vi "Get Wheel Type from String.vi"(10 "dvr (F)":bool, 11 "wheel type":string) -> (3 "data type":variant)   [LabVIEW 2017, in "NI_Robotics_Steering Class Types.lvlib"]
uses:
  <vilib>/robotics/Steering/Class Type Definitions/NI_Robotics_Steering Class Types.lvlib
  <vilib>/robotics/Steering/Class Type Definitions/Wheel.ctl
  <vilib>/robotics/Steering/Wheel/NI_Robotics_Wheel.lvclass
  <vilib>/robotics/Steering/Class Type Definitions/Wheel DVR.ctl
  <vilib>/robotics/Steering/Class Type Definitions/Fixed Wheel.ctl
  <vilib>/robotics/Steering/Fixed Wheel/NI_Robotics_Fixed Wheel.lvclass
  <vilib>/robotics/Steering/Class Type Definitions/Fixed Wheel DVR.ctl
  <vilib>/robotics/Steering/Class Type Definitions/Steering Wheel.ctl
  <vilib>/robotics/Steering/Steering Wheel/NI_Robotics_Steering Wheel.lvclass
  <vilib>/robotics/Steering/Class Type Definitions/Steering Wheel DVR.ctl
  <vilib>/robotics/Steering/Class Type Definitions/Caster Wheel.ctl
  <vilib>/robotics/Steering/Caster Wheel/NI_Robotics_Caster Wheel.lvclass
  <vilib>/robotics/Steering/Class Type Definitions/Caster Wheel DVR.ctl
  <vilib>/robotics/Steering/Class Type Definitions/Mecanum Wheel.ctl
  <vilib>/robotics/Steering/Mecanum Wheel/NI_Robotics_Mecanum Wheel.lvclass
  <vilib>/robotics/Steering/Class Type Definitions/Mecanum Wheel DVR.ctl
  <vilib>/robotics/Steering/Class Type Definitions/Omnidirectional Wheel.ctl
  <vilib>/robotics/Steering/Omnidirectional Wheel/NI_Robotics_Omnidirectional Wheel.lvclass
  <vilib>/robotics/Steering/Class Type Definitions/Omnidirectional Wheel DVR.ctl
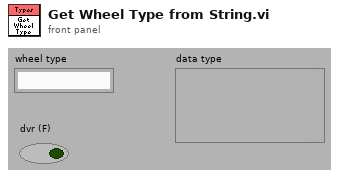
[diagram p1: front panel]
types:
  T1 = typedef "NI_Robotics_Steering Class Types.lvlib/Wheel.ctl" = refnum<class "NI_Robotics_Wheel.lvclass">
  T2 = typedef "NI_Robotics_Steering Class Types.lvlib/Wheel DVR.ctl" = refnum<data-value>
  T3 = typedef "NI_Robotics_Steering Class Types.lvlib/Fixed Wheel.ctl" = refnum<class "NI_Robotics_Fixed Wheel.lvclass">
  T4 = typedef "NI_Robotics_Steering Class Types.lvlib/Fixed Wheel DVR.ctl" = refnum<data-value>
  T5 = typedef "NI_Robotics_Steering Class Types.lvlib/Steering Wheel.ctl" = refnum<class "NI_Robotics_Steering Wheel.lvclass">
  T6 = typedef "NI_Robotics_Steering Class Types.lvlib/Steering Wheel DVR.ctl" = refnum<data-value>
  T7 = typedef "NI_Robotics_Steering Class Types.lvlib/Caster Wheel.ctl" = refnum<class "NI_Robotics_Caster Wheel.lvclass">
  T8 = typedef "NI_Robotics_Steering Class Types.lvlib/Caster Wheel DVR.ctl" = refnum<data-value>
  T9 = typedef "NI_Robotics_Steering Class Types.lvlib/Mecanum Wheel.ctl" = refnum<class "NI_Robotics_Mecanum Wheel.lvclass">
  T10 = typedef "NI_Robotics_Steering Class Types.lvlib/Mecanum Wheel DVR.ctl" = refnum<data-value>
  T11 = typedef "NI_Robotics_Steering Class Types.lvlib/Omnidirectional Wheel.ctl" = refnum<class "NI_Robotics_Omnidirectional Wheel.lvclass">
  T12 = typedef "NI_Robotics_Steering Class Types.lvlib/Omnidirectional Wheel DVR.ctl" = refnum<data-value>
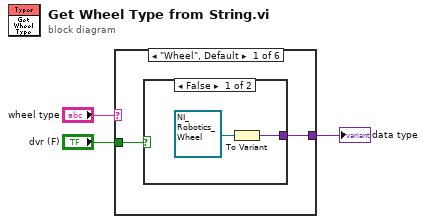
[diagram p0: block diagram]
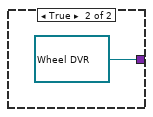
[diagram p2: hidden frame]
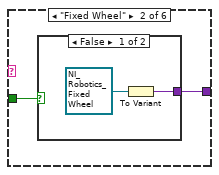
[diagram p3: hidden frame]
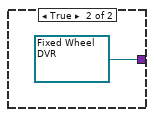
[diagram p4: hidden frame]
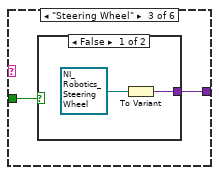
[diagram p5: hidden frame]
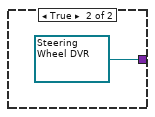
[diagram p6: hidden frame]
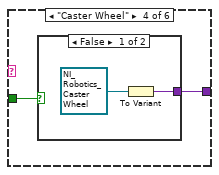
[diagram p7: hidden frame]
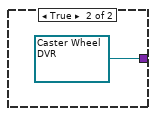
[diagram p8: hidden frame]
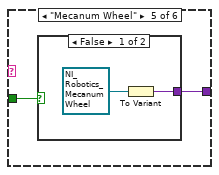
[diagram p9: hidden frame]
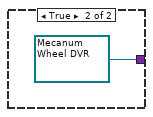
[diagram p10: hidden frame]
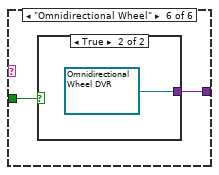
[diagram p11: hidden frame]
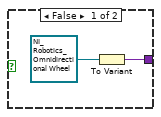
[diagram p12: hidden frame]
diagram:
  n1 = case shown="\"Wheel\", Default" "wheel type" {
    tunnel: "dvr (F)" -> [w5 w10 w15 w20 w25 w30]
    tunnel: [w4 w9 w14 w19 w24 w29] -> w1
    frame "Wheel", Default {
      n2 = case shown="False" w5 {
        tunnel: [w7 T2 refnum ("wheel ref")] -> w4
        frame False {
          n3 = To Variant(anything=T1 refnum ("wheel")) -> (Variant=w7:variant)
        }
        frame True {
        }
      }
    }
    frame "Fixed Wheel" {
      n4 = case shown="False" w10 {
        tunnel: [w12 T4 refnum ("fixed wheel ref")] -> w9
        frame False {
          n5 = To Variant(anything=T3 refnum ("fixed wheel")) -> (Variant=w12:variant)
        }
        frame True {
        }
      }
    }
    frame "Steering Wheel" {
      n6 = case shown="False" w15 {
        tunnel: [w17 T6 refnum ("steering wheel ref")] -> w14
        frame False {
          n7 = To Variant(anything=T5 refnum ("steering wheel")) -> (Variant=w17:variant)
        }
        frame True {
        }
      }
    }
    frame "Caster Wheel" {
      n8 = case shown="False" w20 {
        tunnel: [w22 T8 refnum ("caster wheel ref")] -> w19
        frame False {
          n9 = To Variant(anything=T7 refnum ("caster wheel")) -> (Variant=w22:variant)
        }
        frame True {
        }
      }
    }
    frame "Mecanum Wheel" {
      n10 = case shown="False" w25 {
        tunnel: [w27 T10 refnum ("mecanum wheel ref")] -> w24
        frame False {
          n11 = To Variant(anything=T9 refnum ("mecanum wheel")) -> (Variant=w27:variant)
        }
        frame True {
        }
      }
    }
    frame "Omnidirectional Wheel" {
      n12 = case shown="True" w30 {
        tunnel: [w32 T12 refnum ("omnidirectional wheel ref")] -> w29
        frame False {
          n13 = To Variant(anything=T11 refnum ("omnidirectional wheel")) -> (Variant=w32:variant)
        }
        frame True {
        }
      }
    }
  }
  "data type" <- w1
